vi "ConvertStringtoArray.vi"(7 "delimiter (Tab)":string, 10 "Filter":string) -> (2 "Array":string[](array[string]))   [LabVIEW 2022 SP3]
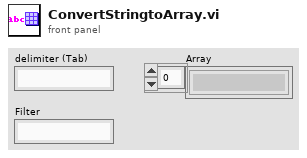
[diagram p1: front panel]
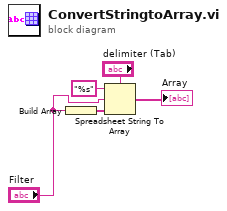
[diagram p0: block diagram]
diagram:
  n1 = Build Array("Filter") -> (w4:string[])
  n2 = Spreadsheet String To Array(delimiter (Tab)="delimiter (Tab)", format string="%s", spreadsheet string="Filter", array type (2D Dbl)=w4) -> (array=→"Array":string[])
